vi "Sum.vi"(10 "Reflections to ignore":cluster{"Numeric":u64, "Numeric":u64}, 11 "Proto In":refnum<class "Group.lvclass">) -> (2 "Reflections":cluster{"Numeric":u64, "Numeric":u64}, 3 "Numeric":u64)   [LabVIEW 2020, in "Group.lvclass"]
uses:
  Group.lvclass
  Group.lvclass/Group.ctl
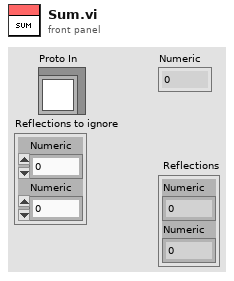
[diagram p1: front panel]
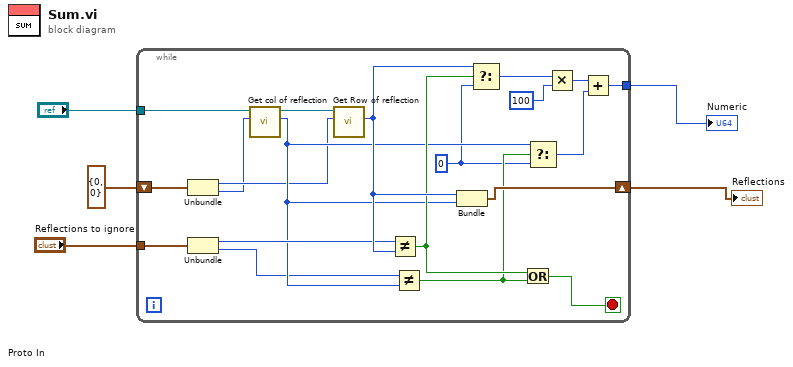
[diagram p0: block diagram]
diagram:
  n1 = while {
    tunnel: [w25] -> w5
    tunnel: "Proto In" -> [w24]
    tunnel: "Reflections to ignore" -> [w19]
    shift-right: [w22] -> w3
    shift-left: cluster{"Numeric":u64, "Numeric":u64} {"Numeric"=0, "Numeric"=0} ("output cluster") -> [w11]
    stop <- w12 stop-if-true
    w6 = u64 0 ("f")
    n2 = Unbundle(w11) -> ("Numeric"=w10:u64, "Numeric"=w9:u64)
    n3 = Unbundle(w19) -> ("Numeric"=w16:u64, "Numeric"=w13:u64)
    n4 = call "Get col of reflection.vi"("Start point"=w9, "Proto in"=w24) -> ("Numeric"=w14:u64, "Proto out"=w23:refnum<class "Group.lvclass">)  [unwired: 7 in, 1 out]
    n5 = call "Get Row of reflection.vi"("Start point"=w10, "Proto in"=w23) -> ("Numeric"=w18:u64)  [unwired: 7 in, 2 out]
    n6 = Not Equal?(x=w16, y=w18) -> (x != y?=w17:bool)
    n7 = Not Equal?(x=w13, y=w14) -> (x != y?=w15:bool)
    n8 = Bundle("Numeric"=w18, "Numeric"=w14) -> (w22:cluster{"Numeric":u64, "Numeric":u64})  [unwired: 1 in]
    n9 = Select(t=w18, s=w17, f=w6) -> (s? t:f=w8:u64)
    n10 = Or(x=w17, y=w15) -> (x .or. y?=w12:bool)
    n11 = Select(t=w14, s=w15, f=w6) -> (s? t:f=w7:u64)
    n12 = Multiply(x=w8, y=u64 100) -> (x*y=w21:u64)
    n13 = Add(x=w21, y=w7) -> (x+y=w25:u64)
  }
  "Numeric" <- w5
  "Reflections" <- w3
